vi "CS_cRIO-PB_DP-Slave_ModuleProperties.vi"(0 "FPGA VI Reference":T2, 11 "Error":errorcluster) -> (4 "FPGA VI Reference out":T2, 8 "cRIO-PB Module":T1 {"ModuleID" format="%.0x"; "VendorID" format="%.0x"}, 15 "Error out":errorcluster)   [LabVIEW 2013, in "dynamic profibus.lvlib"]
uses:
  dynamic profibus.lvlib
  CS_cRIO-PB_DP-Slave_FPGA-Reference.ctl
  <vilib>/rvi/interface/common/niFpgaWaitOnOcc.vi
  <vilib>/Utility/error.llb/Error Cluster From Error Code.vi
  <vilib>/rvi/errors/niLvFpgaAdjustHostInterfaceError.vi
  <vilib>/rvi/interface/nirviReadWriteControl/nirviReadWriteControl.xnode
  NiFpgaLv.dll
  <vilib>/rvi/interface/Simulation/niFpgaSimulationCallBeginRW.vi
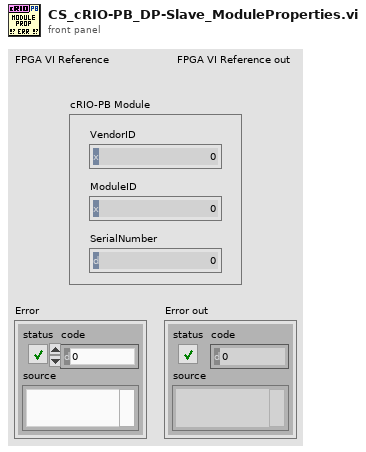
[diagram p1: front panel]
types:
  T1 = cluster{"VendorID":u16, "ModuleID":u16, "SerialNumber":u32}
  T2 = typedef "dynamic profibus.lvlib/CS_cRIO-PB_DP-Slave_FPGA-Reference.ctl" = refnum<k20>
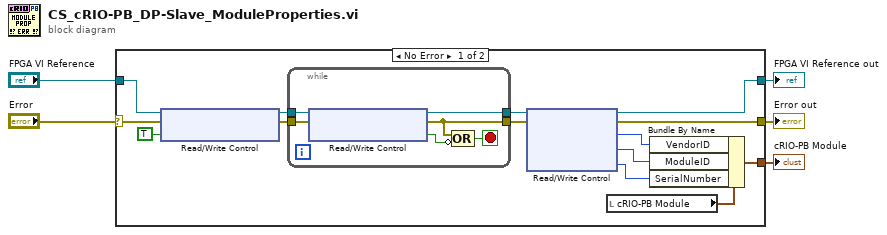
[diagram p0: block diagram]
diagram:
  n1 = case shown="No Error" "Error" {
    selector: "Error" -> [w9 w26]
    tunnel: "FPGA VI Reference" -> [w8 w27]
    tunnel: [w6 w27] -> w3
    tunnel: [w7 w26] -> w2
    tunnel: [w10 _] -> w1
    frame No Error {
      n2 = xnode "Read/Write Control"("FPGA VI Reference In"=w8, "error in"=w9, "cRIO-PB Properties"=TRUE ("GetData")) -> ("FPGA VI Reference Out"=w18:T2, "error out"=w19:errorcluster)
      n3 = while {
        tunnel: w19 -> [w25]
        tunnel: w18 -> [w21]
        tunnel: [w22] -> w17
        tunnel: [w20] -> w16
        stop <- w23 stop-if-true
        n4 = xnode "Read/Write Control"("FPGA VI Reference In"=w21, "error in"=w25) -> ("FPGA VI Reference Out"=w20:T2, "error out"=w22:errorcluster, "cRIO-PB Properties"=w24:bool)
        n5 = Compound Arithmetic op=OR(w22, invert w24) -> (w23:bool)
      }
      n6 = xnode "Read/Write Control"("FPGA VI Reference In"=w16, "error in"=w17) -> ("FPGA VI Reference Out"=w6:T2, "error out"=w7:errorcluster, "VendorID"=w13:u16, "ModuleID"=w12:u16, "SerialNumber"=w11:u32)
      n7 = local read "cRIO-PB Module"() -> (w14:T1)
      n8 = Bundle By Name(cluster=w14, "VendorID"=w13, "ModuleID"=w12, "SerialNumber"=w11) -> (w10:T1)
    }
    frame Error {
    }
  }
  "FPGA VI Reference out" <- w3
  "Error out" <- w2
  "cRIO-PB Module" <- w1
